vi "NI VeriStand - Close Workspace Manager Reference.vi"(8 "error in (no error)":errorcluster, 11 "WorkspaceManager":T1) -> (0 "error out":errorcluster)   [LabVIEW 2020, in "NI_VS Workspace ExecutionAPI.lvlib"]
doc: "Closes an open reference to the workspace manager on the VeriStand Gateway. Use this VI to close each workspace manager reference that you open with the Open Workspace Manager Reference VI."
uses:
  <vilib>/NI VeriStand/Execution/Workspace/NI_VS Workspace ExecutionAPI.lvlib
  <vilib>/NI VeriStand/Execution/Workspace/WorkspaceAPI.ctl
  NationalInstruments.VeriStand.ClientAPI
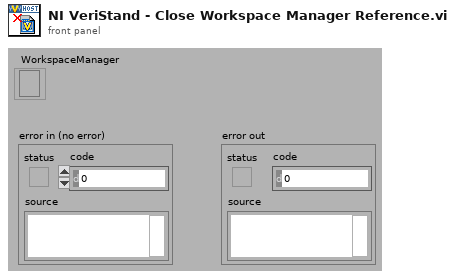
[diagram p1: front panel]
types:
  T1 = typedef "NI_VS Workspace ExecutionAPI.lvlib/WorkspaceAPI.ctl" = refnum<k24>
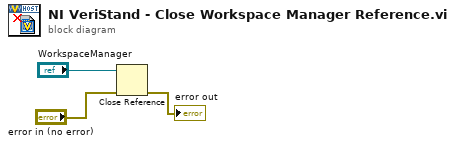
[diagram p0: block diagram]
diagram:
  n1 = Close Reference(reference="WorkspaceManager", error in (no error)="error in (no error)") -> (error out=→"error out":errorcluster)
